vi "String_Detect & Remove specified strings.vi"(6 "Replace with (default is empty)":string, 9 "Array of illegal characters or whole words":string[](array[string]), 11 "Input string":string) -> (1 "Illegal string detected":bool, 3 "String with illegal elements removed":string)   [LabVIEW 2013]
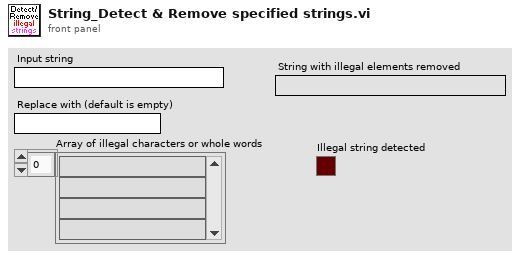
[diagram p1: front panel]
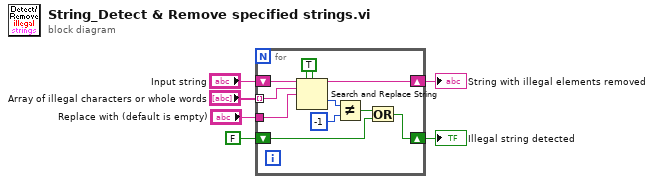
[diagram p0: block diagram]
diagram:
  n1 = for {
    tunnel: "Array of illegal characters or whole words" -> [w16] mode=indexing
    shift-right: [w12] -> w4
    shift-left: "Input string" -> [w13]
    shift-right: [w9] -> w2
    shift-left: FALSE -> [w8]
    tunnel: "Replace with (default is empty)" -> [w7]
    w11 = TRUE ("replace all? (F)")
    n2 = Search and Replace String(replace all?=w11, case sensitive?=w11, input string=w13, search string=w16, replace string=w7) -> (result string=w12:string, offset past replacement=w14:i32)  [unwired: 3 in, 2 out]
    n3 = Not Equal?(x=w14, y=-1) -> (x != y?=w10:bool)
    n4 = Or(x=w10, y=w8) -> (x .or. y?=w9:bool)
  }
  "String with illegal elements removed" <- w4
  "Illegal string detected" <- w2
